vi "get_all.vi"(8 "error in (no error)":errorcluster, 11 "Headers in":refnum<class "Headers.lvclass">) -> (0 "error out":errorcluster, 1 "headers":string, 2 "headers":cluster{"name":string, "value":string}[](array[cluster]), 3 "Headers in":refnum<class "Headers.lvclass">)   [LabVIEW 2020, in "reqwest.lvlib" / "Headers.lvclass"]
uses:
  Headers.lvclass
  Headers.lvclass/Headers.ctl
  reqwest.lvlib
  lv_reqwest_32.dll
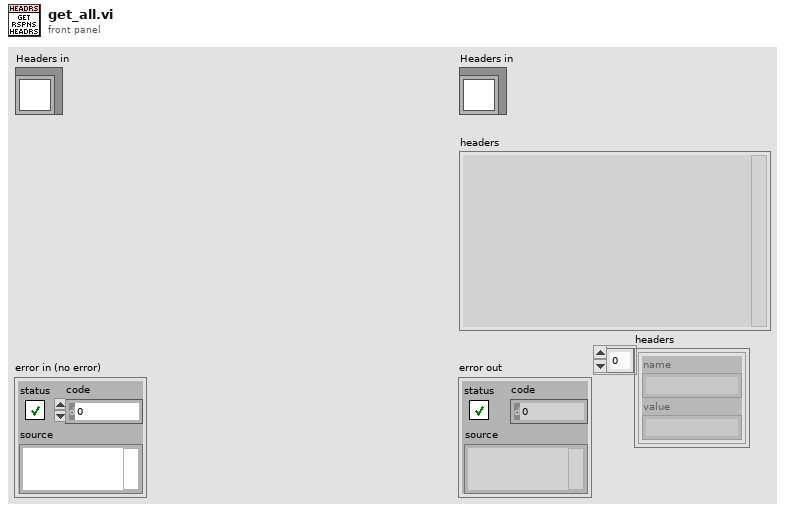
[diagram p1: front panel]
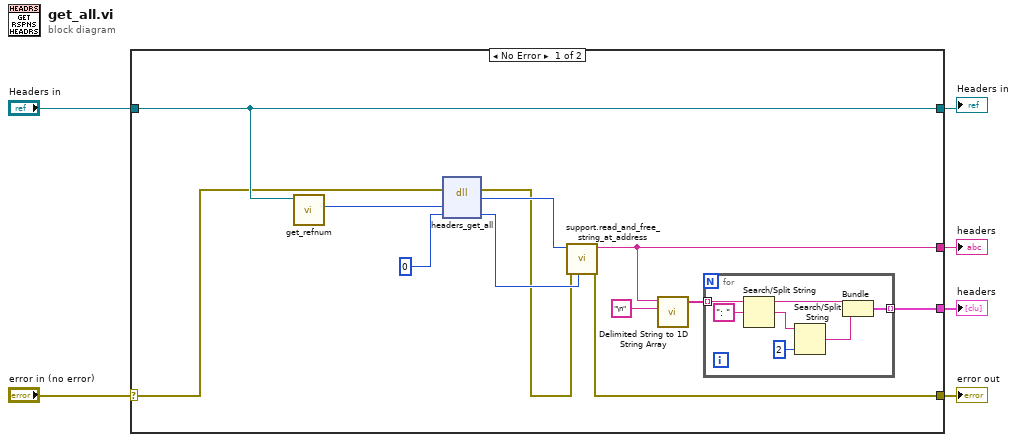
[diagram p0: block diagram]
diagram:
  n1 = case shown="No Error" "error in (no error)" {
    selector: "error in (no error)" -> [w16 w26]
    tunnel: "Headers in" -> [w18 w27]
    tunnel: [w11 w26] -> w3
    tunnel: [w18 w27] -> w4
    tunnel: [w9 _] -> w2
    tunnel: [w10 _] -> w1
    frame No Error {
      n2 = call "get_refnum.vi"("Headers in"=w18) -> ("ref"=w15:u64)  [unwired: 10 in]
      n3 = dll-call lib="C:/Projects/reqwest-rs-labview/lv_src/lv_reqwest_*.*" fn="headers_get_all"(error in=w16, "request_id"=w15, "num_bytes"=u32 0) -> (error out=w12:errorcluster, "string_ptr"=w14:u64, "num_bytes"=w13:u32)  [unwired: 3 in, 1 out]
      n4 = call "support.read_and_free_string_at_address.vi"("string_length"=w13, "error in (no error)"=w12, "string_ptr"=w14) -> ("error out"=w11:errorcluster, "string"=w9:string)  [unwired: 7 in]
      n5 = call <vilib>:"Delimited String to 1D String Array.vi"("delimiter"="\n", "delimited string"=w9) -> ("string array"=w7:string[])  [unwired: 9 in]
      n6 = for {
        tunnel: w7 -> [w25] mode=indexing
        tunnel: [w22] -> w10 mode=indexing
        n7 = Search/Split String(string=w25, search string/char (-)=": ") -> (substring before match=w23:string, match + rest of string=w20:string)  [unwired: 1 in, 1 out]
        n8 = Search/Split String(string=w20, offset (0)=2) -> (match + rest of string=w19:string)  [unwired: 1 in, 2 out]
        n9 = Bundle("String"=w23, "String"=w19) -> (w22:cluster{"String":string, "String":string})  [unwired: 1 in]
      }
    }
    frame Error {
    }
  }
  "error out" <- w3
  "Headers in" <- w4
  "headers" <- w2
  "headers" <- w1
